vi "Write Controls.vi"(9 "Wiring Rules":T1(array[ring]), 10 "Controls[]":refnum<vi>[](array[refnum]), 11 "Message Scripter in":refnum<class "Message Scripter.lvclass">) -> (3 "Message Scripter out":refnum<class "Message Scripter.lvclass">)   [LabVIEW 2020, in "Message Maker.lvlib" / "Message Scripter.lvclass"]
uses:
  Message Scripter.lvclass
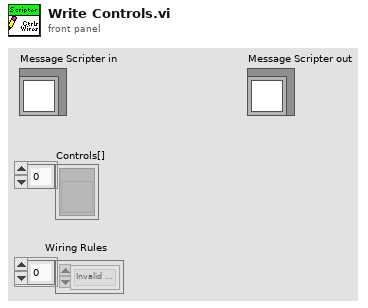
[diagram p1: front panel]
types:
  T1 = enum16{"Invalid Wire Rule", "Required", "Recommended", "Optional", "Dynamic Dispatch"}[]
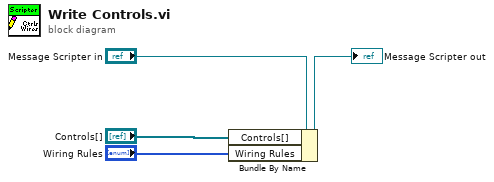
[diagram p0: block diagram]
diagram:
  n1 = Bundle By Name(cluster="Message Scripter in", "Controls[]"="Controls[]", "Wiring Rules"="Wiring Rules") -> (→"Message Scripter out":refnum<class "Message Scripter.lvclass">)
